vi "ReadScan1.vi"(8 "error in (no error)":errorcluster, 9 "number":u32, 10 "Data In":refnum<vi>, 11 "Data In":T3) -> (0 "error out":errorcluster, 1 "Next State":T2=enum."State1", 2 "States":T1=enum."Initialize", 3 "Data Out":T3, 5 "Data Out":refnum<vi>)   [LabVIEW 2014]
doc: "Use this template to build a standard state machine design pattern. Each state executes code and determines which state to transition to. Contrast this design pattern with the User Interface Event Handler pattern, in which code executes in response to user actions. Contrast this design pattern also with the Queued Message Handler pattern, in which each message handling code can queue zero or more new messages.\nNote: This template does not contain the most recent programming guidelines recommended by National Instruments. For a complete, project-based implementation of the Standard State Machine pattern, use the Create Project dialog box instead of this template."
uses:
  Data1.ctl
  Payjson.ctl
  Wait Scan States.ctl
  State.ctl
  ReadScan1States.ctl
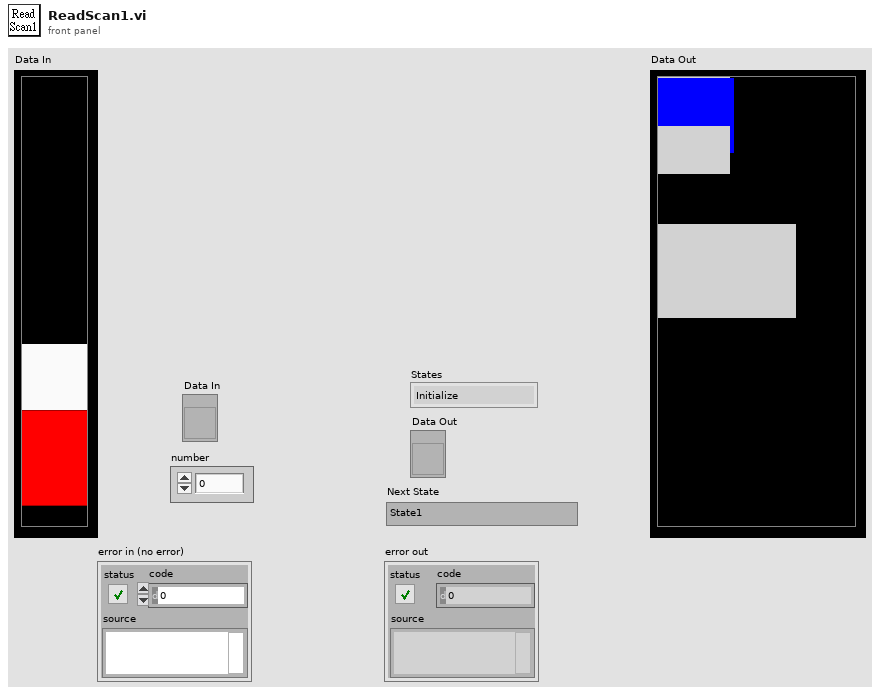
[diagram p1: front panel]
types:
  T1 = typedef "State.ctl" = enum16{"int", "Initalize0", "Initialize", "Wait for Scan", "State 1", "State 2", "NG", "NG1", "OK", "OKNG", "OKNG1", "Exit"}
  T2 = typedef "Wait Scan States.ctl" = enum16{"Initialize", "State1", "Stop"}
  T3 = typedef "Data1.ctl" = cluster{"Date":string, "BarCode1":string, "BarCode2":string, "BarCode3":string, "Message":string, "OK Count":u16, "NG Count":u16, "Total Count":u16, "ModelData":string[][], "OK&NG":bool, "COM1":refnum<visa-resource-name>, "COM2":refnum<visa-resource-name>, "IO":i32, "Time":u32, "TCP":refnum<k5>, "TCP 2":refnum<k5>, "COM1 2":refnum<visa-resource-name>, "CheckNum":string, "BarCode1_1":string, "BarCode2_1":string, "BarCode3_1":string, "日期":string, "機種":string, "機號":string, "商品條碼1":string, "OK_1":string, "OK":string, "NG":string, "NG_1":string, "Total":string, "Total_1":string, "ClaerTime":u32, "Pjson":T4, "LotNo":string[], "CheckParsArray":string[], "BarCode4":string, "BarCode4_1":string, "商品條碼2":string, "BarCode5":string, "BarCode5_1":string, "商品條碼3":string, "ReScanNG":i32, "NGTimeCT":u32}
  T4 = typedef "Payjson.ctl" = cluster{"DEPT":string, "LINE":string, "STANO":string, "WORKNO":string, "PRODSN":string, "COMPNTID":string, "COMPNTLOT":string, "COMPNTSN":string, "USEDQTY":i16, "OPDATE":string, "OPUSER":string, "RECVDATE":string, "MMODU":string}[]
  T5 = typedef "ReadScan1States.ctl" = enum16{"Initialize", "Init2", "Step1", "Step2", "Step3", "Step4", "One", "Two", "Three", "Four", "Five", "End", "Stop"}
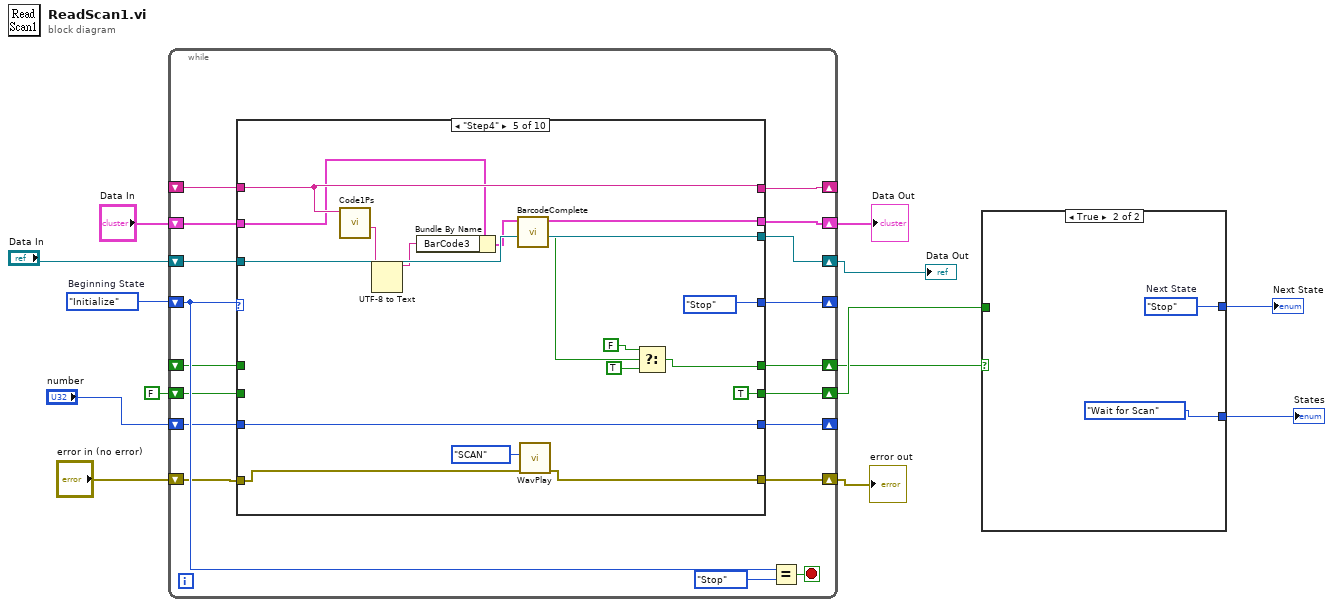
[diagram p0: block diagram]
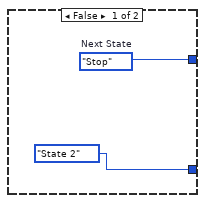
[diagram p2: hidden frame]
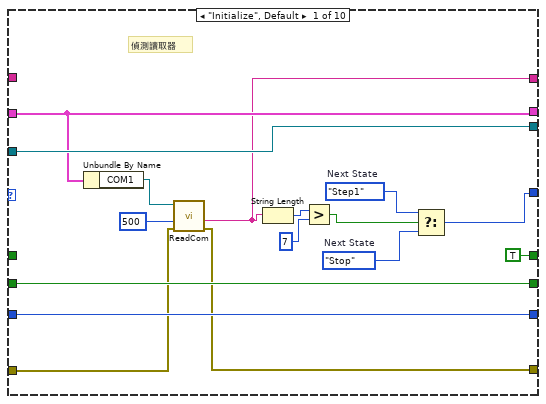
[diagram p3: hidden frame]
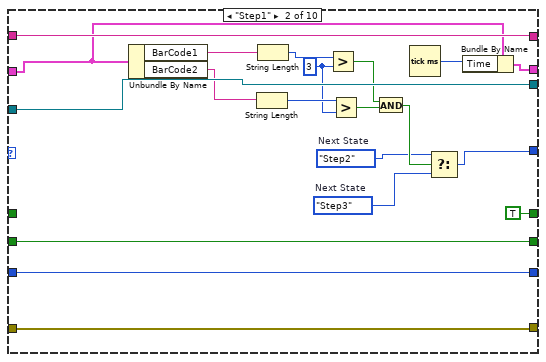
[diagram p4: hidden frame]
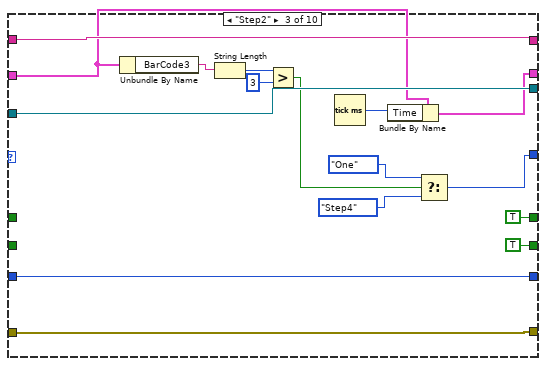
[diagram p5: hidden frame]
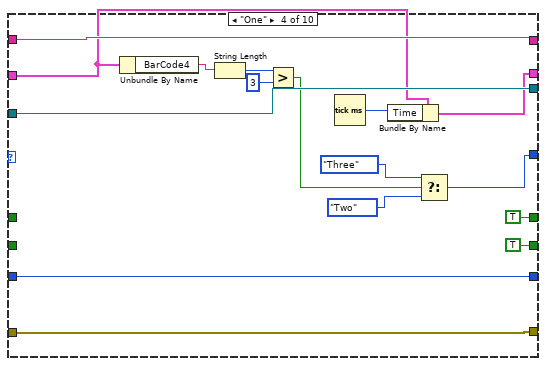
[diagram p6: hidden frame]
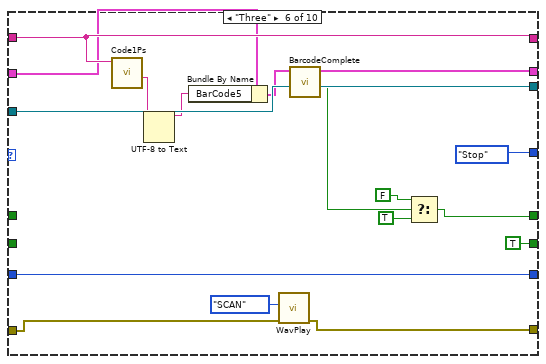
[diagram p7: hidden frame]
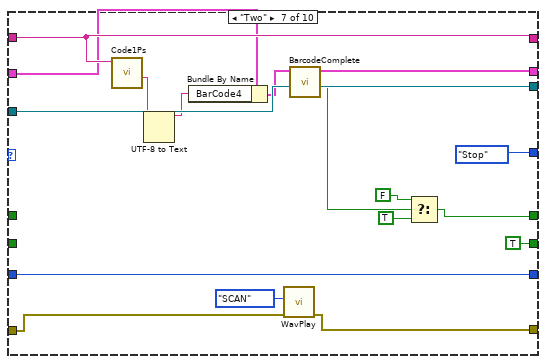
[diagram p8: hidden frame]
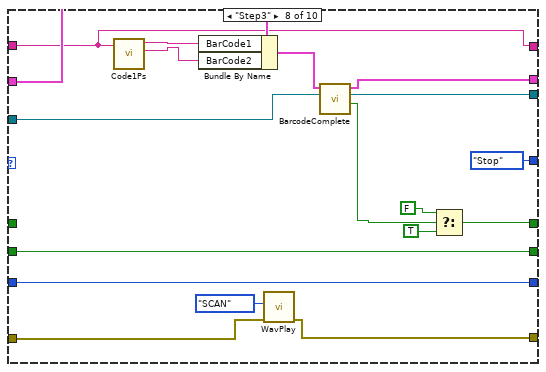
[diagram p9: hidden frame]
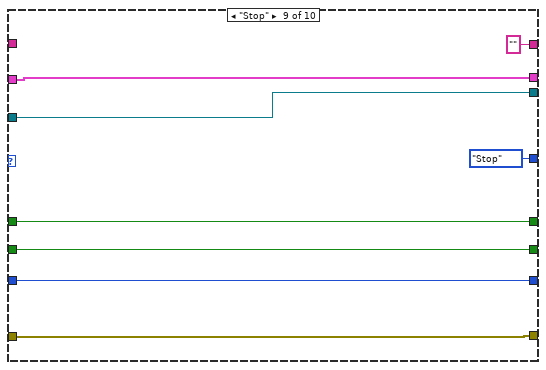
[diagram p10: hidden frame]
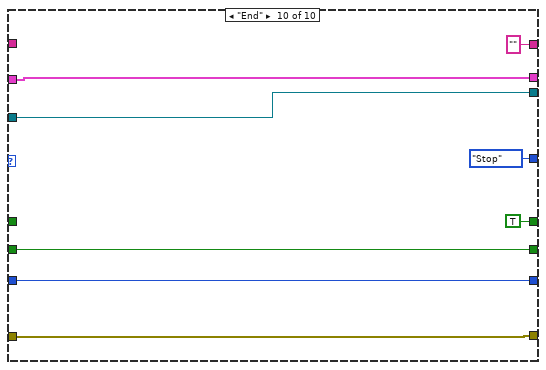
[diagram p11: hidden frame]
diagram:
  w13 = ReadScan1States."Initialize"  # Beginning State
  n1 = while {
    shift-right: [w28] -> _
    shift-left: w13 -> [w29]
    shift-right: [w23] -> w11
    shift-left: "Data In" -> [w26]
    shift-right: [w22] -> w9
    shift-left: "error in (no error)" -> [w27]
    shift-right: [w24] -> _
    shift-left: _ -> [w25]
    shift-right: [w21] -> w5
    shift-left: FALSE -> [w20]
    shift-right: [w18] -> w3
    shift-left: "Data In" -> [w19]
    shift-right: [w16] -> _
    shift-left: "number" -> [w17]
    shift-right: [w15] -> w1
    shift-left: _ -> [w14]
    stop <- w31 stop-if-true
    n2 = case shown="\"Step4\"" w29 {
      tunnel: [w45 w52 w69 w85 ReadScan1States."Stop" ("Next State") ReadScan1States."Stop" ("Next State") ReadScan1States."Stop" ("Next State") ReadScan1States."Stop" ("Next State") ReadScan1States."Stop" ("Next State") ReadScan1States."Stop" ("Next State")] -> w28
      tunnel: w27 -> [w36 w63 w82 w98 w102 w119 w136 w153 w172 w180]
      tunnel: w26 -> [w33 w50 w74 w90 w115 w132 w149 w161 w173 w181]
      tunnel: w25 -> [_ w51 w83 w99 w116 w133 w150 w160 _ _]
      tunnel: [w32 w51 w83 w99 w116 w133 w150 w160 "" ""] -> w24
      tunnel: [w33 w49 w73 w89 w105 w122 w139 w158 w173 w181] -> w23
      tunnel: [w35 w63 w82 w98 w101 w118 w135 w152 w172 w180] -> w22
      tunnel: [w44 w67 TRUE TRUE TRUE TRUE TRUE w166 w171 w179] -> w21
      tunnel: w20 -> [w44 w67 _ _ _ _ _ w166 w171 w179]
      tunnel: w19 -> [w43 w64 w80 w96 w112 w129 w146 w165 w170 w178]
      tunnel: [w43 w64 w80 w96 w112 w129 w146 w165 w170 w178] -> w18
      tunnel: w17 -> [w42 w66 w79 w95 w111 w128 w145 w164 w169 w177]
      tunnel: [w42 w66 w79 w95 w111 w128 w145 w164 w169 w177] -> w16
      tunnel: [TRUE TRUE TRUE ("f") TRUE ("f") w108 w125 w142 w154 w168 TRUE] -> w15
      tunnel: w14 -> [_ _ _ _ _ _ _ _ w168 _]
      frame "Initialize", Default {
        w47 = ReadScan1States."Step1"  # Next State
        w46 = ReadScan1States."Stop"  # Next State
        # "偵測讀取器"
        n3 = Unbundle By Name(w33) -> ("COM1"=w38:refnum<visa-resource-name>)
        n4 = call "ReadCom.vi"("error in (no error)"=w36, "delay before read (ms)"=u32 500, "Com In"=w38) -> ("error out"=w35:errorcluster, "Response"=w32:string)  [unwired: 5 in, 2 out]
        n5 = String Length(string=w32) -> (length=w40:i32)
        n6 = Greater?(x=w40, y=7) -> (0:w34:bool)
        n7 = Select(t=w47, s=w34, f=w46) -> (s? t:f=w45:T5)
      }
      frame "Step1" {
        w53 = ReadScan1States."Step2"  # Next State
        w58 = 3 ("y")
        w54 = ReadScan1States."Step3"  # Next State
        n8 = Unbundle By Name(w50) -> ("BarCode1"=w62:string, "BarCode2"=w61:string)
        n9 = String Length(string=w61) -> (length=w59:i32)
        n10 = String Length(string=w62) -> (length=w60:i32)
        n11 = Greater?(x=w60, y=w58) -> (0:w56:bool)
        n12 = Greater?(x=w59, y=w58) -> (0:w57:bool)
        n13 = And(x=w56, y=w57) -> (x .and. y?=w55:bool)
        n14 = Tick Count (ms)() -> (millisecond timer value=w48:u32)
        n15 = Select(t=w53, s=w55, f=w54) -> (s? t:f=w52:T5)
        n16 = Bundle By Name(cluster=w50, "Time"=w48) -> (w49:T3)
      }
      frame "Step2" {
        n17 = Unbundle By Name(w74) -> ("BarCode3"=w76:string)
        n18 = String Length(string=w76) -> (length=w78:i32)
        n19 = Greater?(x=w78, y=3) -> (0:w71:bool)
        n20 = Tick Count (ms)() -> (millisecond timer value=w75:u32)
        n21 = Bundle By Name(cluster=w74, "Time"=w75) -> (w73:T3)
        n22 = Select(t=ReadScan1States."One" ("Next State"), s=w71, f=ReadScan1States."Step4" ("Next State")) -> (s? t:f=w69:T5)
      }
      frame "One" {
        n23 = Unbundle By Name(w90) -> ("BarCode4"=w92:string)
        n24 = String Length(string=w92) -> (length=w94:i32)
        n25 = Greater?(x=w94, y=3) -> (0:w87:bool)
        n26 = Tick Count (ms)() -> (millisecond timer value=w91:u32)
        n27 = Bundle By Name(cluster=w90, "Time"=w91) -> (w89:T3)
        n28 = Select(t=ReadScan1States."Three" ("Next State"), s=w87, f=ReadScan1States."Two" ("Next State")) -> (s? t:f=w85:T5)
      }
      frame "Step4" {
        n29 = call "Code1Ps.vi"("Code1 In"=w116) -> ("紙箱號碼"=w104:string)  [unwired: 8 in, 2 out]
        n30 = UTF-8 to Text(11:w104) -> (3:w103:string)  [unwired: 2 in, 1 out]
        n31 = Bundle By Name(cluster=w115, "BarCode3"=w103) -> (w110:T3)
        n32 = call "BarcodeComplete.vi"("Data In"=w110) -> ("Complete"=w106:bool, "Data Out"=w105:T3)  [unwired: 9 in]
        n33 = call "WavPlay.vi"("error in (no error)"=w102, "OkNg"=enum16{"OK", "NG", "NG1", "SCAN"}."SCAN") -> ("error out"=w101:errorcluster)  [unwired: 9 in]
        n34 = Select(t=FALSE, s=w106, f=TRUE) -> (s? t:f=w108:bool)
      }
      frame "Three" {
        n35 = call "Code1Ps.vi"("Code1 In"=w133) -> ("紙箱號碼"=w121:string)  [unwired: 8 in, 2 out]
        n36 = UTF-8 to Text(11:w121) -> (3:w120:string)  [unwired: 2 in, 1 out]
        n37 = Bundle By Name(cluster=w132, "BarCode5"=w120) -> (w127:T3)
        n38 = call "WavPlay.vi"("error in (no error)"=w119, "OkNg"=enum16{"OK", "NG", "NG1", "SCAN"}."SCAN") -> ("error out"=w118:errorcluster)  [unwired: 9 in]
        n39 = call "BarcodeComplete.vi"("Data In"=w127) -> ("Complete"=w123:bool, "Data Out"=w122:T3)  [unwired: 9 in]
        n40 = Select(t=FALSE, s=w123, f=TRUE) -> (s? t:f=w125:bool)
      }
      frame "Two" {
        n41 = call "Code1Ps.vi"("Code1 In"=w150) -> ("紙箱號碼"=w138:string)  [unwired: 8 in, 2 out]
        n42 = UTF-8 to Text(11:w138) -> (3:w137:string)  [unwired: 2 in, 1 out]
        n43 = Bundle By Name(cluster=w149, "BarCode4"=w137) -> (w144:T3)
        n44 = call "WavPlay.vi"("error in (no error)"=w136, "OkNg"=enum16{"OK", "NG", "NG1", "SCAN"}."SCAN") -> ("error out"=w135:errorcluster)  [unwired: 9 in]
        n45 = call "BarcodeComplete.vi"("Data In"=w144) -> ("Complete"=w140:bool, "Data Out"=w139:T3)  [unwired: 9 in]
        n46 = Select(t=FALSE, s=w140, f=TRUE) -> (s? t:f=w142:bool)
      }
      frame "Step3" {
        n47 = call "Code1Ps.vi"("Code1 In"=w160) -> ("機種代號"=w163:string, "機種名"=w162:string)  [unwired: 8 in, 1 out]
        n48 = Bundle By Name(cluster=w161, "BarCode1"=w162, "BarCode2"=w163) -> (w159:T3)
        n49 = call "WavPlay.vi"("error in (no error)"=w153, "OkNg"=enum16{"OK", "NG", "NG1", "SCAN"}."SCAN") -> ("error out"=w152:errorcluster)  [unwired: 9 in]
        n50 = call "BarcodeComplete.vi"("Data In"=w159) -> ("Complete"=w155:bool, "Data Out"=w158:T3)  [unwired: 9 in]
        n51 = Select(t=FALSE, s=w155, f=TRUE) -> (s? t:f=w154:bool)
      }
      frame "Stop" {
      }
      frame "End" {
      }
    }
    n52 = Equal?(x=w29, y=ReadScan1States."Stop" ("States")) -> (x = y?=w31:bool)
  }
  "Data Out" <- w11
  "error out" <- w9
  "Data Out" <- w3
  n53 = case shown="True" w1 {
    tunnel: [w185 w187] -> w8
    tunnel: [State."State 2" ("States") State."Wait for Scan" ("States")] -> w7
    tunnel: w5 -> [_ _]
    frame False {
      w185 = Wait_Scan_States."Stop"  # Next State
    }
    frame True {
      w187 = Wait_Scan_States."Stop"  # Next State
    }
  }
  "Next State" <- w8
  "States" <- w7
